vi "ai labview.vi"   [LabVIEW 2021]
uses:
  Terminal.ctl
types:
  T1 = typedef "bd.ctl" = cluster{"Nodes":refnum<class "Node.lvclass">[], "Wires":T2[], "name":string, "UUID":string}
  T2 = typedef "wire.ctl" = cluster{"id":string, "from":string, "to":string}
  T3 = typedef "Terminal.ctl" = cluster{"id":string, "name":string, "terminal":refnum<vi>}
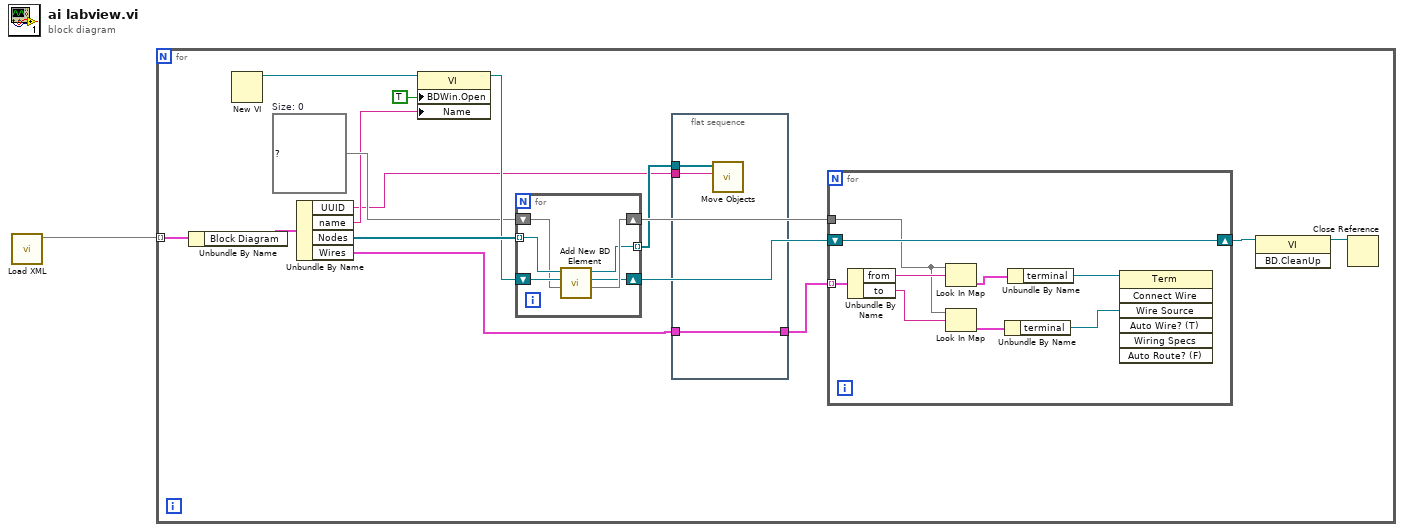
[diagram p0: block diagram]
diagram:
  n1 = call "Load XML.vi"() -> ("Map"=w1:map{string, T1})  [unwired: 11 in]
  n2 = for {
    tunnel: w1 -> [w17] mode=indexing
    w11 = map{string, T3} {}  # Size: 0
    n3 = Unbundle By Name(w17) -> ("Block Diagram"=w16:T1)
    n4 = New VI() -> (3:w14:refnum<vi>)  [unwired: 7 in, 1 out]
    n5 = Unbundle By Name(w16) -> ("UUID"=w4:string, "name"=w6:string, "Nodes"=w15:refnum<class "Node.lvclass">[], "Wires"=w3:T2[])
    n6 = property class="VI"(reference=w14, "BDWin.Open"=TRUE ("Block Diagram Window:Open"), "Name"=w6) -> (reference out=w12:refnum<vi>)  [unwired: 1 in, 1 out]
    n7 = for {
      tunnel: w15 -> [w34] mode=indexing
      shift-right: [w31] -> w10
      shift-left: w12 -> [w35]
      shift-right: [w32] -> w9
      shift-left: w11 -> [w33]
      tunnel: [w30] -> w5 mode=indexing
      n8 = call "Add New BD Element.vi"("Map in"=w33, "vi refnum in"=w35, "Node in"=w34) -> ("Map out"=w32:map{string, T3}, "vi refnum out"=w31:refnum<vi>, "Node out"=w30:refnum<class "Node.lvclass">)  [unwired: 6 in]
    }
    n9 = flat-sequence {
      tunnel: w5 -> [w20]
      tunnel: w4 -> [w19]
      tunnel: w3 -> [w18]
      tunnel: [w18] -> w2
      frame #0 {
        n10 = call "Move Objects.vi"("BD UUID"=w19, "Array"=w20) -> ()  [unwired: 10 in]
      }
    }
    n11 = for {
      tunnel: w2 -> [w29] mode=indexing
      shift-right: [w28] -> w8
      shift-left: w10 -> [w28]
      tunnel: w9 -> [w26]
      n12 = Unbundle By Name(w29) -> ("from"=w27:string, "to"=w25:string)
      n13 = Look In Map(map=w26, key=w27) -> (value=w24:T3)  [unwired: 1 in, 1 out]
      n14 = Look In Map(map=w26, key=w25) -> (value=w23:T3)  [unwired: 1 in, 1 out]
      n15 = Unbundle By Name(w23) -> ("terminal"=w21:refnum<vi>)
      n16 = Unbundle By Name(w24) -> ("terminal"=w22:refnum<vi>)
      n17 = invoke class="Term" method="Connect Wire"(reference=w22, "Wire Source"=w21) -> ()  [unwired: 5 in, 7 out]
    }
    n18 = invoke class="VI" method="BD.CleanUp"(reference=w8) -> (reference out=w7:refnum<vi>)  [unwired: 2 in, 2 out]
    n19 = Close Reference(reference=w7) -> ()  [unwired: 1 in, 1 out]
  }
